vi "BLT-STATIC-CONFIG.vi"() -> ()   [LabVIEW 2018]
uses:
  Type Defs/Sensor Data.ctl
  Type Defs/Boxcar.ctl
panel:
  out "?":string="27.79 °C"
  out "?":string="27.79 °C"
  out "45% 2":string="27.79 °C"
  out "45%":string="27.79 °C"
  in  "Box cooler":bool
  out "NewVal":bool
  out "Ready To Fire Flag":bool
  out "Firing State":string[](array[string])=["System Is Not Armed", "", "", "", "", " "]
  in  "Arm Flag":bool
  in  "Sample Rate (secs)":u32=1000
  out "Burn Time\nCountdown (secs)":string="0.00"
  out "Boxcar Data":T1={"AI Sensor Data"={"Sensor Array"=[{"Description"="PT LOX Tank", "Last Reading"="1.37", "Coefs"=[0.0, 0.0], "Eng Units"="Psig"}, {"Description"="P3 - Fuel Tank Pressure", "Last Reading"="0.24", "Coefs"=[0.0, 5000.0], "Eng Units"="psig"}, {"Description"="P1 - Chamber Pressure", "Last Reading"="68.57", "Coefs"=[0.0, 5000.0], "Eng Units"="psig"}, {"Description"="Not Used", "Last Reading"="88.17", "Coefs"=[0.0, 0.0], "Eng Units"="psig"}, {"Description"="P5- DOME Reg.", "Last Reading"="1995.18", "Coefs"=[0.0, 5000.0], "Eng Units"="psig"}, {"Description"="Not Use", "Last Reading"="30.30", "Coefs"=[0.0, 0.0], "Eng Units"="psig"}, {"Description"="P4- High Pressure Tank", "Last Reading"="45.96", "Coefs"=[0.0, 10000.0], "Eng Units"="psig"}, {"Description"="P7 - Gnd High Pressure", "Last Reading"="1989.04", "Coefs"=[0.0, 10000.0], "Eng Units"="psig"}, {"Description"="P6 - GHE Fill Pressure", "Last Reading"="9918.82", "Coefs"=[0.0, 5000.0], "Eng Units"="psig"}, {"Description"="P8 - Pneumatics Pressure", "Last Reading"="9988.56", "Coefs"=[0.0, 5000.0], "Eng Units"="psig"}, {"Description"="Not Used", "Last Reading"="9997.25", "Coefs"=[0.0, 0.0], "Eng Units"=""}, {"Description"="Not Used", "Last Reading"="9988.56", "Coefs"=[0.0, 0.0], "Eng Units"=""}, {"Description"="Not Used", "Last Reading"="9948.58", "Coefs"=[0.0, 0.0], "Eng Units"=""}, {"Description"="Not Used", "Last Reading"="9973.45", "Coefs"=[0.0, 0.0], "Eng Units"=""}, {"Description"="Not Used", "Last Reading"="9964.45", "Coefs"=[0.0, 0.0], "Eng Units"=""}, {"Description"="PT High Press", "Last Reading"="9.16", "Coefs"=[0.0, 0.0], "Eng Units"="Psig"}, {"Description"="QD Sep Indication", "Last Reading"="2374.97", "Coefs"=[0.0, 1.0], "Eng Units"="On/Off"}, {"Description"="Lift Off Indicator", "Last Reading"="2375.24", "Coefs"=[0.0, 1.0], "Eng Units"="On/Off"}, {"Description"="Main Valve Open Indicator", "Last Reading"="2376.46", "Coefs"=[0.0, 1.0], "Eng Units"="On/Off"}, {"Description"="Main Valve Closed Indicator", "Last Reading"="2376.23", "Coefs"=[0.0, 1.0], "Eng Units"="On/Off"}, {"Description"="Load Cell 1 - Veh Gross Weight", "Last Reading"="2374.97", "Coefs"=[-122.0, 8333.3], "Eng Units"="lbf"}, {"Description"="Load Cell 2 - - Veh Gross Weight", "Last Reading"="2374.97", "Coefs"=[0.0, 8333.33], "Eng Units"="lbf"}, {"Description"="Not Used", "Last Reading"="2374.97", "Coefs"=[0.0, 0.0], "Eng Units"=""}, {"Description"="Not Used", "Last Reading"="2374.97", "Coefs"=[0.0, 0.0], "Eng Units"=""}, {"Description"="PT Fuel Tank", "Last Reading"="10.72", "Coefs"=[], "Eng Units"="Psig"}, {"Description"="", "Last Reading"="2401.98", "Coefs"=[], "Eng Units"=""}, {"Description"="PT Dome Set", "Last Reading"="0", "Coefs"=[], "Eng Units"="Psig"}, {"Description"="", "Last Reading"="2402.71", "Coefs"=[], "Eng Units"=""}, {"Description"="", "Last Reading"="2402.21", "Coefs"=[], "Eng Units"=""}, {"Description"="", "Last Reading"="2401.71", "Coefs"=[], "Eng Units"=""}, {"Description"="", "Last Reading"="2401.48", "Coefs"=[], "Eng Units"=""}, {"Description"="", "Last Reading"="2400.99", "Coefs"=[], "Eng Units"=""}]}, "TC Array"=[27.792357874999993, 27.792357874999993, 27.792357874999993, 27.792357874999993, 27.792357874999993, 27.792357874999993, 27.792357874999993, 1369.6815, 1369.6815, 1369.6815, 1369.6815, 1369.6815, 1369.6815, 1369.6815]}
  out "?":string="3.07 psig"
  out "Log Refnum":refnum<file>
  out "Log Epoch":u32
  out "Log Number":i32=8
  in  "Data Log Flag":bool
  out "File Path":path
  out "Eng Data & Units":string[](array[string])
  out "TC String Array":string[](array[string])=["27.79 °C", "27.79 °C", "27.79 °C", "27.79 °C", "27.79 °C", "27.79 °C", "27.79 °C", "1369.68 °C", "1369.68 °C", "1369.68 °C", "1369.68 °C", "1369.68 °C", "1369.68 °C", "1369.68 °C"]
  in  "Data Log Button":bool
  in  "Sequence Abort":bool
  out "Igniter Abort":bool
  out "Elapsed Time":u32=10554
  in  "Auto Sequence":bool
  in  "Auto Sequence Flag":bool
  out "Epoch":u32=5746771
  out "Countdown (secs)":i32
  in  "MV Open Start":dbl
  in  "Burn Time":dbl=10.0
  in  "Igniter Start":dbl=-3.0
  in  "Countdown":dbl=-10.0
  in  "Igniter Minimum\nTemp (°C)":dbl=200.0
  in  "Auto Switch":bool=TRUE
  out "?":string="1369.68 °C"
  out "Thermometer 2":dbl(slide)=1369.6815 scale=0.0..1000.0
  out "Thermometer":dbl(slide)=1369.6815 scale=0.0..1000.0
  out "Igniter Temp (°C)":string="1369.68 °C"
  out "?":string="27.79 °C"
  out "30%":string="27.79 °C"
  out "QD Sep Indicator":bool=TRUE
  out "Liftoff Indicator":bool=TRUE
  out "MV Closed Ind":bool
  out "MV Open Ind":bool
  out "?":string="0.13 lbf"
  out "?":string="0.32 psig"
  out "?":string="-4.62 psig"
  out "Dome Set PT":string="-1.58 psig"
  out "High Press PT":string="-1.56 psig"
  out "?":string="-1.17 psig"
  out "FUEL Tank PT":string="-1.03 psig"
  in  "High Press":bool
  in  "High Press Vent":bool
  in  "MV Open":bool
  in  "MV Closed":bool
  out "LOX Tank PT":string="-1.67 psig"
  in  "Remote QD Sep":bool
  in  "GHe Fill":bool
  in  "Igniter Pwr":bool
  in  "Dome Reg":bool
  in  "Dome Vent":bool
  in  "Fuel Vent":bool
  in  "LOX Vent":bool
  out "Relay States":bool[](array[boolean])
  in  "stop":bool
  in  "AI Sensor Data":T2={"Sensor Array"=[{"Description"="PT LOX Tank", "Last Reading"="1.37", "Coefs"=[0.0, 0.0], "Eng Units"="Psig"}, {"Description"="P3 - Fuel Tank Pressure", "Last Reading"="0.24", "Coefs"=[0.0, 5000.0], "Eng Units"="psig"}, {"Description"="P1 - Chamber Pressure", "Last Reading"="68.57", "Coefs"=[0.0, 5000.0], "Eng Units"="psig"}, {"Description"="Not Used", "Last Reading"="88.17", "Coefs"=[0.0, 0.0], "Eng Units"="psig"}, {"Description"="P5- DOME Reg.", "Last Reading"="1995.18", "Coefs"=[0.0, 5000.0], "Eng Units"="psig"}, {"Description"="Not Use", "Last Reading"="30.30", "Coefs"=[0.0, 0.0], "Eng Units"="psig"}, {"Description"="P4- High Pressure Tank", "Last Reading"="45.96", "Coefs"=[0.0, 10000.0], "Eng Units"="psig"}, {"Description"="P7 - Gnd High Pressure", "Last Reading"="1989.04", "Coefs"=[0.0, 10000.0], "Eng Units"="psig"}, {"Description"="P6 - GHE Fill Pressure", "Last Reading"="9918.82", "Coefs"=[0.0, 5000.0], "Eng Units"="psig"}, {"Description"="P8 - Pneumatics Pressure", "Last Reading"="9988.56", "Coefs"=[0.0, 5000.0], "Eng Units"="psig"}, {"Description"="Not Used", "Last Reading"="9997.25", "Coefs"=[0.0, 0.0], "Eng Units"=""}, {"Description"="Not Used", "Last Reading"="9988.56", "Coefs"=[0.0, 0.0], "Eng Units"=""}, {"Description"="Not Used", "Last Reading"="9948.58", "Coefs"=[0.0, 0.0], "Eng Units"=""}, {"Description"="Not Used", "Last Reading"="9973.45", "Coefs"=[0.0, 0.0], "Eng Units"=""}, {"Description"="Not Used", "Last Reading"="9964.45", "Coefs"=[0.0, 0.0], "Eng Units"=""}, {"Description"="PT High Press", "Last Reading"="9.16", "Coefs"=[0.0, 0.0], "Eng Units"="Psig"}, {"Description"="QD Sep Indication", "Last Reading"="2374.97", "Coefs"=[0.0, 1.0], "Eng Units"="On/Off"}, {"Description"="Lift Off Indicator", "Last Reading"="2375.24", "Coefs"=[0.0, 1.0], "Eng Units"="On/Off"}, {"Description"="Main Valve Open Indicator", "Last Reading"="2376.46", "Coefs"=[0.0, 1.0], "Eng Units"="On/Off"}, {"Description"="Main Valve Closed Indicator", "Last Reading"="2376.23", "Coefs"=[0.0, 1.0], "Eng Units"="On/Off"}, {"Description"="Load Cell 1 - Veh Gross Weight", "Last Reading"="2374.97", "Coefs"=[-122.0, 8333.3], "Eng Units"="lbf"}, {"Description"="Load Cell 2 - - Veh Gross Weight", "Last Reading"="2374.97", "Coefs"=[0.0, 8333.33], "Eng Units"="lbf"}, {"Description"="Not Used", "Last Reading"="2374.97", "Coefs"=[0.0, 0.0], "Eng Units"=""}, {"Description"="Not Used", "Last Reading"="2374.97", "Coefs"=[0.0, 0.0], "Eng Units"=""}, {"Description"="PT Fuel Tank", "Last Reading"="10.72", "Coefs"=[], "Eng Units"="Psig"}, {"Description"="", "Last Reading"="2401.98", "Coefs"=[], "Eng Units"=""}, {"Description"="PT Dome Set", "Last Reading"="0", "Coefs"=[], "Eng Units"="Psig"}, {"Description"="", "Last Reading"="2402.71", "Coefs"=[], "Eng Units"=""}, {"Description"="", "Last Reading"="2402.21", "Coefs"=[], "Eng Units"=""}, {"Description"="", "Last Reading"="2401.71", "Coefs"=[], "Eng Units"=""}, {"Description"="", "Last Reading"="2401.48", "Coefs"=[], "Eng Units"=""}, {"Description"="", "Last Reading"="2400.99", "Coefs"=[], "Eng Units"=""}]}
  # "CSULB Launch Team Control System"
  # "Questions regrads this system please direct them to Thanh Truc Le truclee126@gmail.com"
  # "Autosequence\n Parameters"
  # "TOP"
  # "TOP"
  # "CENTER"
  # "CENTER"
  # "BOTTOM"
  # "BOTTOM"
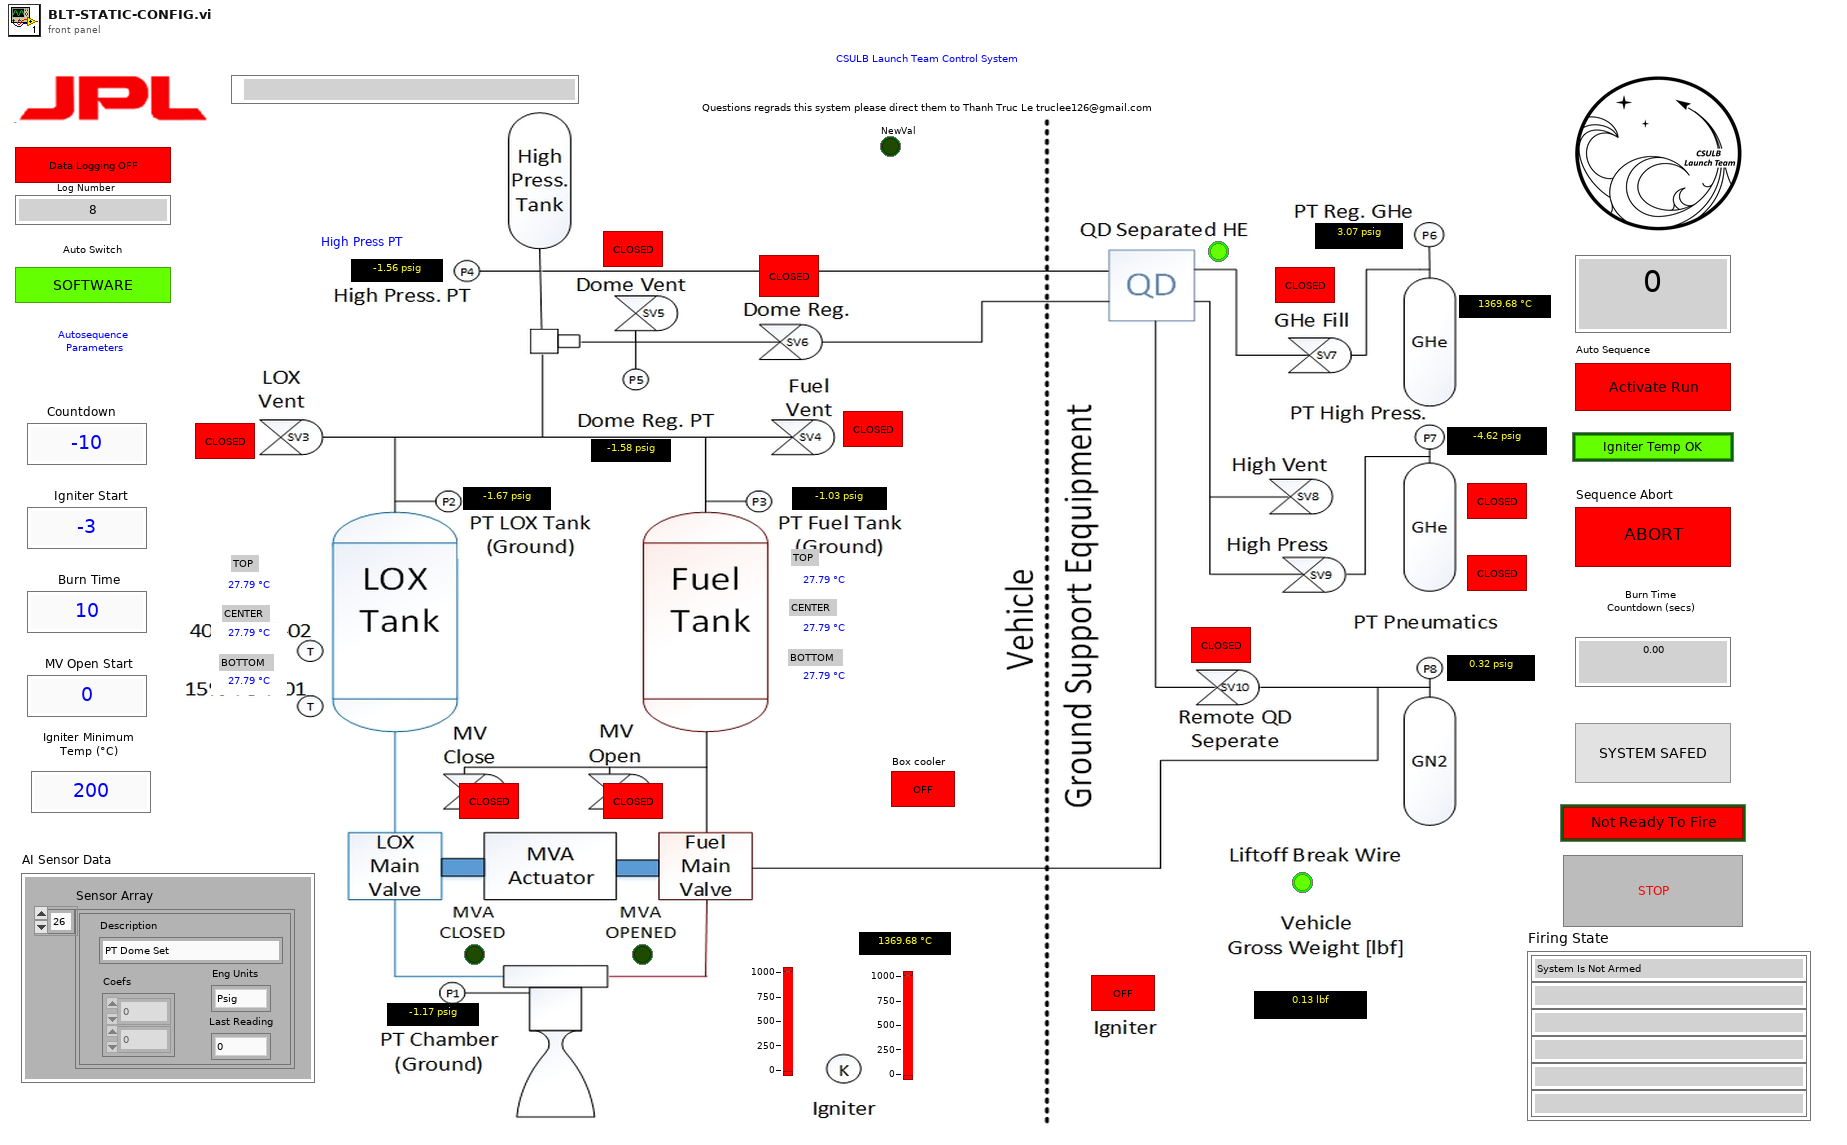
[diagram p1: front panel]
types:
  T1 = typedef "Boxcar.ctl" = cluster{"AI Sensor Data":T2, "TC Array":dbl[]}
  T2 = typedef "Sensor Data.ctl" = cluster{"Sensor Array":cluster{"Description":string, "Last Reading":string, "Coefs":dbl[], "Eng Units":string}[]}
  T3 = cluster{"Description":string, "Last Reading":string, "Coefs":dbl[], "Eng Units":string}[]
  T4 = enum16{"open", "replace", "create", "open or create", "replace or create", "replace or create with confirmation"}
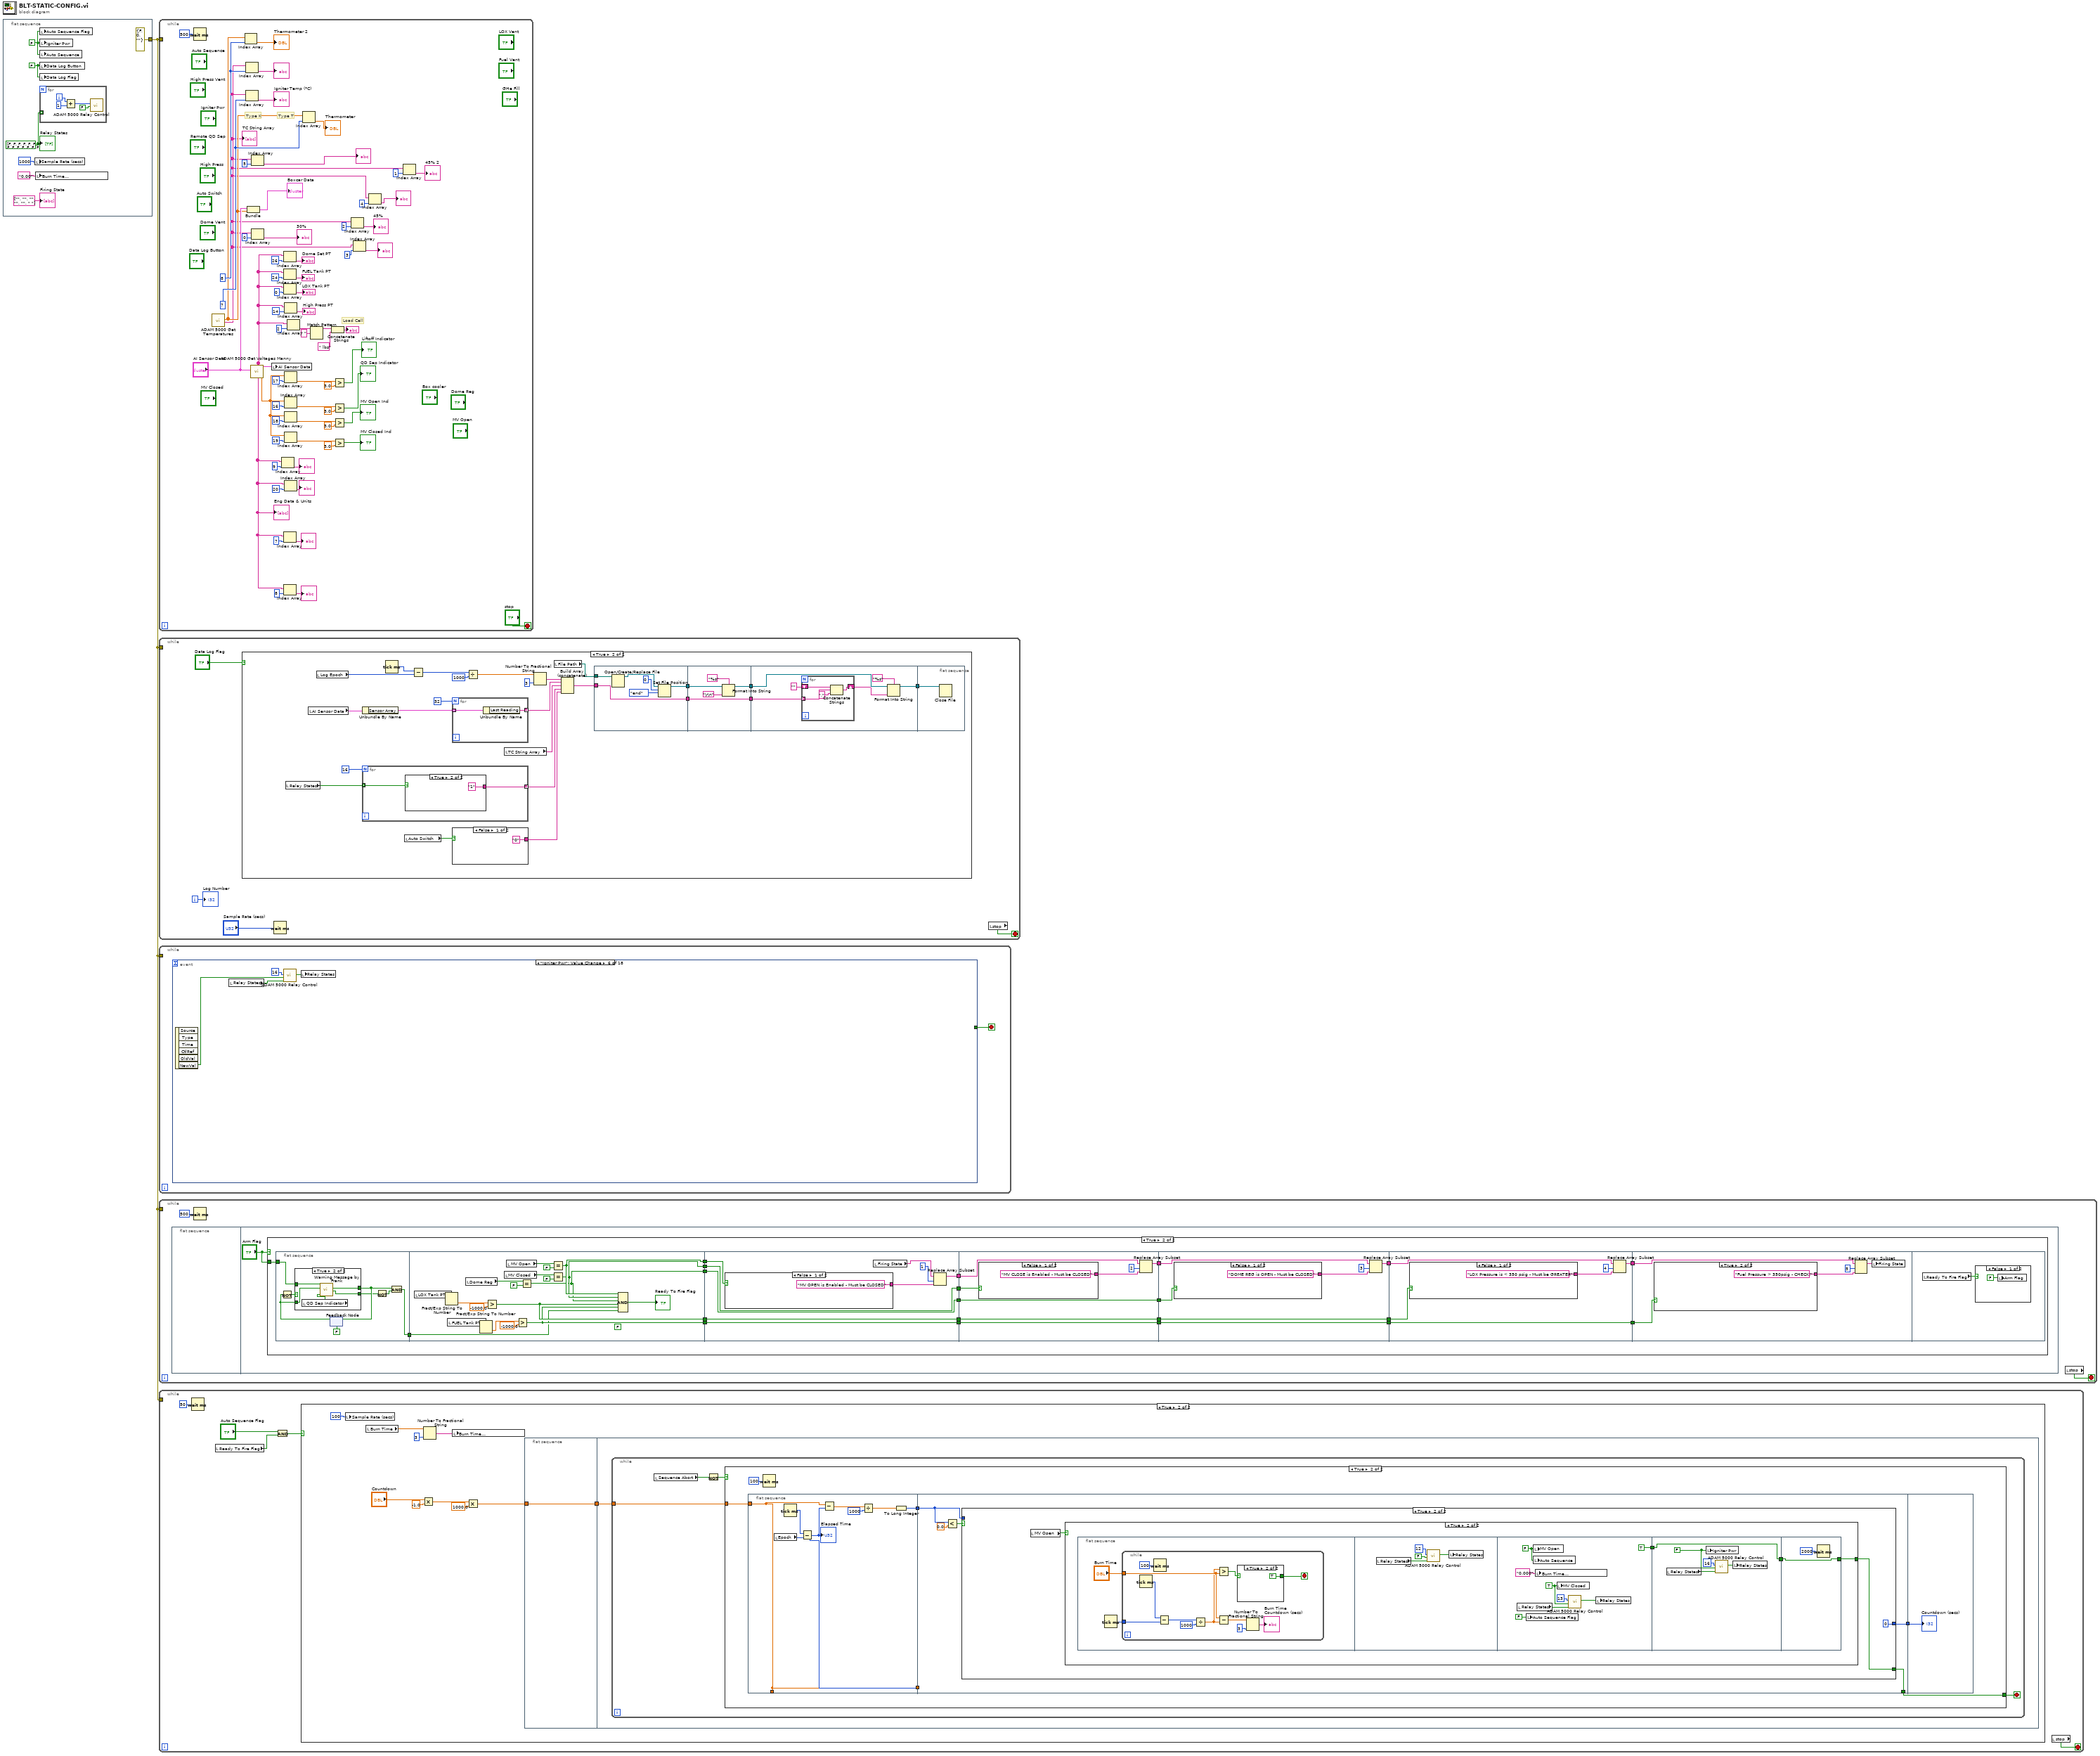
[diagram p0: block diagram]
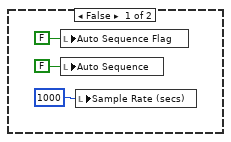
[diagram p2: hidden frame]
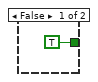
[diagram p3: hidden frame]
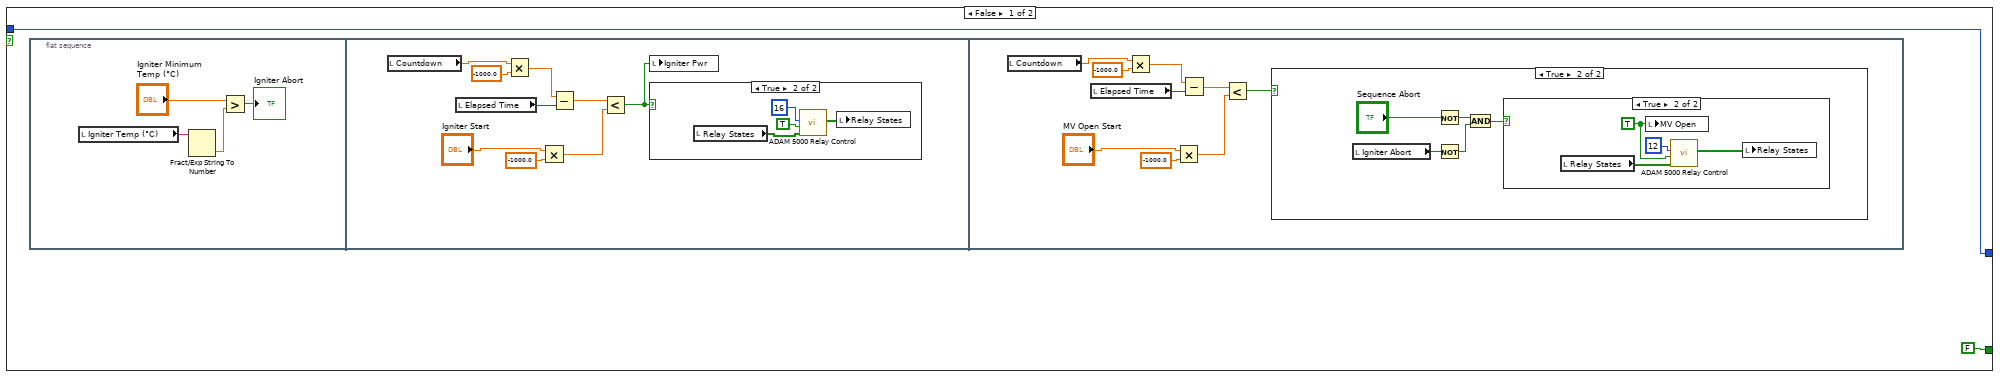
[diagram p4: hidden frame]
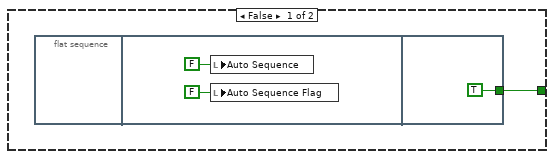
[diagram p8: hidden frame]
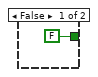
[diagram p9: hidden frame]
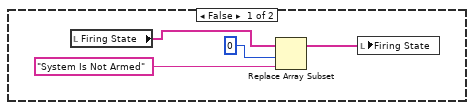
[diagram p10: hidden frame]
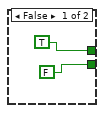
[diagram p11: hidden frame]
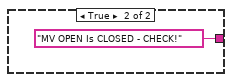
[diagram p12: hidden frame]
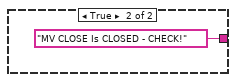
[diagram p13: hidden frame]
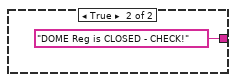
[diagram p14: hidden frame]
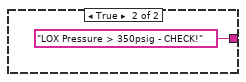
[diagram p15: hidden frame]
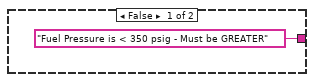
[diagram p16: hidden frame]
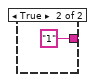
[diagram p19: hidden frame]
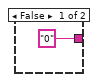
[diagram p20: hidden frame]
diagram:
  n1 = flat-sequence {
    tunnel: [errorcluster {"status"=FALSE, "code"=0, "source"=""} ("error constant")] -> w1
    frame #0 {
      w5 = FALSE ("Data Lof Flag")
      w6 = FALSE ("Auto Sequence Flag")
      w7 = bool[] [FALSE, FALSE, FALSE, FALSE, FALSE, FALSE, FALSE, FALSE, FALSE, FALSE, FALSE, FALSE, FALSE, FALSE, FALSE, FALSE]
      n2 = local write "Sample Rate (secs)"(u32 1000 ("Sample Rate (secs)")) -> ()
      n3 = local write "Burn Time\nCountdown (secs)"("0.00" ("Burn Time\nCountdown (secs)")) -> ()
      n4 = local write "Auto Sequence Flag"(w6) -> ()
      n5 = local write "Igniter Pwr"(w6) -> ()
      n6 = local write "Auto Sequence"(w6) -> ()
      n7 = local write "Data Log Button"(w5) -> ()
      n8 = local write "Data Log Flag"(w5) -> ()
      n9 = for {
        tunnel: w7 -> [_] mode=indexing
        i -> [w12]
        n10 = Add(x=w12, y=1) -> (x+y=w10:i32)
        n11 = call "ADAM 5000 Relay Control.vi"("State"=FALSE, "Relay # (1=1st relay)"=w10) -> ()  [unwired: 9 in, 1 out]
      }
      "Relay States" <- w7
      "Firing State" <- string[] ["", "", "", "", "", " "]
    }
  }
  n12 = while {
    tunnel: w1 -> [_]
    stop <- "stop" stop-if-true
    w37 = 7 ("index")
    w34 = 8 ("index")
    # "Load Cell"
    # "Type T"
    # "Type K"
    n13 = Wait (ms)(milliseconds to wait=u32 500) -> ()  [unwired: 1 out]
    n14 = call "ADAM 5000 Get Temperatures.vi"() -> ("TC String Array"=w16:string[], "TC Array"=w28:dbl[])  [unwired: 10 in]
    "TC String Array" <- w16
    n15 = Index Array(array=w28, index=w34) -> (element=→"Thermometer 2":dbl)
    n16 = Index Array(array=w16, index=w34) -> (element=→"?":string)
    n17 = Index Array(array=w16, index=w37) -> (element=→"Igniter Temp (°C)":string)
    n18 = Bundle("AI Sensor Data"="AI Sensor Data", "TC Array"=w28) -> (→"Boxcar Data":cluster{"AI Sensor Data":T2, "TC Array":dbl[]})  [unwired: 1 in]
    n19 = call "ADAM 5000 Get Voltages Manny.vi"("AI Sensor Data"="AI Sensor Data") -> ("Master Raw Data Vdc"=w43:dbl[], "AI Sensor Data Out"=w75:T2, "Eng Data & Units"=w30:string[])  [unwired: 5 in, 3 out]
    "Eng Data & Units" <- w30
    n20 = Index Array(array=w16, index=5) -> (element=→"?":string)
    n21 = Index Array(array=w16, index=0) -> (element=→"30%":string)
    n22 = local write "AI Sensor Data"(w75) -> ()
    n23 = Index Array(array=w30, index=9) -> (element=→"?":string)
    n24 = Index Array(array=w30, index=26) -> (element=→"Dome Set PT":string)
    n25 = Index Array(array=w30, index=24) -> (element=→"FUEL Tank PT":string)
    n26 = Index Array(array=w30, index=7) -> (element=→"?":string)
    n27 = Index Array(array=w30, index=0) -> (element=→"LOX Tank PT":string)
    n28 = Index Array(array=w30, index=8) -> (element=→"?":string)
    n29 = Index Array(array=w30, index=14) -> (element=→"High Press PT":string)
    n30 = Index Array(array=w43, index=17) -> (element=w50:dbl)
    n31 = Index Array(array=w43, index=16) -> (element=w45:dbl)
    n32 = Index Array(array=w43, index=18) -> (element=w58:dbl)
    n33 = Index Array(array=w43, index=19) -> (element=w54:dbl)
    n34 = Index Array(array=w30, index=20) -> (element=→"?":string)
    n35 = Index Array(array=w30, index=2) -> (element=w22:string)
    n36 = Index Array(array=w28, index=w37) -> (element=→"Thermometer":dbl)
    n37 = Match Pattern(string=w22, regular expression=" ") -> (before substring=w20:string)  [unwired: 1 in, 3 out]
    n38 = Concatenate Strings(w20, " lbs" ("string")) -> (→"?":string)
    n39 = Greater?(x=w50, y=3.0) -> (0:→"Liftoff Indicator":bool)
    n40 = Greater?(x=w45, y=3.0) -> (0:→"QD Sep Indicator":bool)
    n41 = Greater?(x=w58, y=3.0) -> (0:→"MV Open Ind":bool)
    n42 = Greater?(x=w54, y=3.0) -> (0:→"MV Closed Ind":bool)
    n43 = Index Array(array=w16, index=2) -> (element=→"45%":string)
    n44 = Index Array(array=w16, index=3) -> (element=→"?":string)
    n45 = Index Array(array=w16, index=4) -> (element=→"?":string)
    n46 = Index Array(array=w16, index=1) -> (element=→"45% 2":string)
  }
  n47 = while {
    tunnel: w1 -> [_]
    i -> [w79]
    stop <- w81 stop-if-true
    n48 = case shown="True" "Data Log Flag" {
      frame False {
      }
      frame True {
        n49 = local read "Relay States"() -> (w103:bool[])
        n50 = local read "AI Sensor Data"() -> (w105:T2)
        n51 = local read "Log Epoch"() -> (w96:u32)
        n52 = Unbundle By Name(w105) -> ("Sensor Array"=w104:T3)
        n53 = for {
          N: 16 -> [_]
          tunnel: w103 -> [w131] mode=indexing
          tunnel: [w130] -> w99 mode=indexing
          n54 = case shown="True" w131 {
            tunnel: ["0" "1"] -> w130
            frame False {
            }
            frame True {
            }
          }
        }
        n55 = Tick Count (ms)() -> (millisecond timer value=w97:u32)
        n56 = local read "Auto Switch"() -> (w102:bool)
        n57 = Subtract(x=w97, y=w96) -> (x-y=w95:u32)
        n58 = for {
          N: 32 -> [_]
          tunnel: w104 -> [w135] mode=indexing
          tunnel: [w134] -> w101 mode=indexing
          n59 = Unbundle By Name(w135) -> ("Last Reading"=w134:string)
        }
        n60 = case shown="False" w102 {
          tunnel: ["0" "1"] -> w98
          frame False {
          }
          frame True {
          }
        }
        n61 = Divide(x=w95, y=u32 1000) -> (x/y=w93:dbl)
        n62 = local read "TC String Array"() -> (w100:string[])
        n63 = Number To Fractional String(number=w93, precision (6)=i16 3) -> (F-format string=w91:string)  [unwired: 2 in]
        n64 = local read "File Path"() -> (w90:path)
        n65 = Build Array (concatenate)(w91, w101, w100, w99, w98) -> (w89:string[])
        n66 = flat-sequence {
          tunnel: w89 -> [w111]
          tunnel: w90 -> [w110]
          tunnel: [w111] -> w87
          tunnel: [w106] -> w84
          tunnel: [w112] -> w88
          tunnel: w87 -> [w116]
          tunnel: [w116] -> w86
          tunnel: w84 -> [w113]
          tunnel: w88 -> [w119]
          tunnel: w86 -> [w122]
          tunnel: [w117] -> w85
          tunnel: w85 -> [w127]
          frame #0 {
            n67 = Open/Create/Replace File(file path (use dialog)=w110) -> (refnum out=w109:refnum<file>)  [unwired: 5 in, 2 out]
            n68 = Set File Position(offset (in bytes) (0)=i64 0, refnum=w109, from (0:start)=enum16{"start", "end", "current"}."end") -> (refnum out=w106:refnum<file>)  [unwired: 1 in, 1 out]
          }
          frame #1 {
            n69 = Format Into String(format string="%s", initial string=w113, "\r\n") -> (resulting string=w112:refnum<file>)  [unwired: 1 in, 1 out]
          }
          frame #2 {
            n70 = for {
              shift-right: [w124] -> w118
              shift-left: "" -> [w123]
              tunnel: w122 -> [w126] mode=indexing
              n71 = Concatenate Strings(w123, w126, "," ("string")) -> (w124:string)
            }
            n72 = Format Into String(format string="%s", initial string=w119, w118) -> (resulting string=w117:refnum<file>)  [unwired: 1 in, 1 out]
          }
          frame #3 {
            n73 = Close File(refnum=w127) -> ()  [unwired: 1 in, 2 out]
          }
        }
      }
    }
    n74 = Wait (ms)(milliseconds to wait="Sample Rate (secs)") -> ()  [unwired: 1 out]
    n75 = local read "stop"() -> (w81:bool)
    "Log Number" <- w79
  }
  n76 = while {
    tunnel: w1 -> [_]
    stop <- w136 stop-if-true
    n77 = event shown="[5] \"Igniter Pwr\": Value Change" {
      selector: _ -> [_ _ _ _ _ _ _ _ _ _ _ _ _ _ _ _ _ _]
      dyn-events: _ -> [_ _ _ _ _ _ _ _ _ _ _ _ _ _ _ _ _ _]
      timeout: _ -> [_ _ _ _ _ _ _ _ _ _ _ _ _ _ _ _ _ _]
      tunnel: [_ _ _ _ _ _ _ _ w165 _ _ _ _ _ _ _ _ _] -> w136
      event Timeout {
        n78 = event-data() -> ()  [unwired: 1 in, 3 out]
      }
      event "LOX Vent": Value Change {
        n79 = event-data() -> ("NewVal"=w139:bool)  [unwired: 1 in, 5 out]
        n80 = local read "Relay States"() -> (w138:bool[])
        n81 = call "ADAM 5000 Relay Control.vi"("Relay States IN"=w138, "State"=w139, "Relay # (1=1st relay)"=1) -> ("Relay States OUT"=w137:bool[])  [unwired: 8 in]
        n82 = local write "Relay States"(w137) -> ()
      }
      event "Fuel Vent": Value Change {
        n83 = event-data() -> ("NewVal"=w141:bool)  [unwired: 1 in, 5 out]
        n84 = local read "Relay States"() -> (w143:bool[])
        n85 = call "ADAM 5000 Relay Control.vi"("Relay States IN"=w143, "State"=w141, "Relay # (1=1st relay)"=2) -> ("Relay States OUT"=w142:bool[])  [unwired: 8 in]
        n86 = local write "Relay States"(w142) -> ()
      }
      event "Dome Vent": Value Change {
        n87 = event-data() -> ("NewVal"=w145:bool)  [unwired: 1 in, 5 out]
        n88 = local read "Relay States"() -> (w147:bool[])
        n89 = call "ADAM 5000 Relay Control.vi"("Relay States IN"=w147, "State"=w145, "Relay # (1=1st relay)"=6) -> ("Relay States OUT"=w146:bool[])  [unwired: 8 in]
        n90 = local write "Relay States"(w146) -> ()
      }
      event "Dome Reg": Value Change {
        n91 = event-data() -> ("NewVal"=w149:bool)  [unwired: 1 in, 5 out]
        n92 = local read "Relay States"() -> (w151:bool[])
        n93 = call "ADAM 5000 Relay Control.vi"("Relay States IN"=w151, "State"=w149, "Relay # (1=1st relay)"=5) -> ("Relay States OUT"=w150:bool[])  [unwired: 8 in]
        n94 = local write "Relay States"(w150) -> ()
      }
      event "Igniter Pwr": Value Change {
        n95 = event-data() -> ("NewVal"=w153:bool)  [unwired: 1 in, 5 out]
        n96 = local read "Relay States"() -> (w155:bool[])
        n97 = call "ADAM 5000 Relay Control.vi"("Relay States IN"=w155, "State"=w153, "Relay # (1=1st relay)"=16) -> ("Relay States OUT"=w154:bool[])  [unwired: 8 in]
        n98 = local write "Relay States"(w154) -> ()
      }
      event "GHe Fill": Value Change {
        n99 = event-data() -> ("NewVal"=w157:bool)  [unwired: 1 in, 5 out]
        n100 = local read "Relay States"() -> (w159:bool[])
        n101 = call "ADAM 5000 Relay Control.vi"("Relay States IN"=w159, "State"=w157, "Relay # (1=1st relay)"=9) -> ("Relay States OUT"=w158:bool[])  [unwired: 8 in]
        n102 = local write "Relay States"(w158) -> ()
      }
      event "Remote QD Sep": Value Change {
        n103 = event-data() -> ("NewVal"=w161:bool)  [unwired: 1 in, 5 out]
        n104 = local read "Relay States"() -> (w163:bool[])
        n105 = call "ADAM 5000 Relay Control.vi"("Relay States IN"=w163, "State"=w161, "Relay # (1=1st relay)"=10) -> ("Relay States OUT"=w162:bool[])  [unwired: 8 in]
        n106 = local write "Relay States"(w162) -> ()
      }
      event "stop": Value Change {
        n107 = event-data() -> ()  [unwired: 1 in, 6 out]
        n108 = flat-sequence {
          tunnel: [TRUE] -> w165
          frame #0 {
            n109 = Wait (ms)(milliseconds to wait=u32 2000) -> ()  [unwired: 1 out]
          }
          frame #1 {
          }
        }
      }
      event "MV Closed": Value Change {
        n110 = event-data() -> ("NewVal"=w168:bool)  [unwired: 1 in, 5 out]
        n111 = local read "Relay States"() -> (w170:bool[])
        n112 = call "ADAM 5000 Relay Control.vi"("Relay States IN"=w170, "State"=w168, "Relay # (1=1st relay)"=13) -> ("Relay States OUT"=w169:bool[])  [unwired: 8 in]
        n113 = local write "Relay States"(w169) -> ()
      }
      event "High Press Vent": Value Change {
        n114 = event-data() -> ("NewVal"=w172:bool)  [unwired: 1 in, 5 out]
        n115 = local read "Relay States"() -> (w174:bool[])
        n116 = call "ADAM 5000 Relay Control.vi"("Relay States IN"=w174, "State"=w172, "Relay # (1=1st relay)"=15) -> ("Relay States OUT"=w173:bool[])  [unwired: 8 in]
        n117 = local write "Relay States"(w173) -> ()
      }
      event "High Press": Value Change {
        n118 = event-data() -> ("NewVal"=w176:bool)  [unwired: 1 in, 5 out]
        n119 = local read "Relay States"() -> (w178:bool[])
        n120 = call "ADAM 5000 Relay Control.vi"("Relay States IN"=w178, "State"=w176, "Relay # (1=1st relay)"=7) -> ("Relay States OUT"=w177:bool[])  [unwired: 8 in]
        n121 = local write "Relay States"(w177) -> ()
      }
      event "Auto Switch": Value Change {
        n122 = event-data() -> ("NewVal"=w181:bool)  [unwired: 1 in, 5 out]
        n123 = call "Control ETH008 Relay.vi"("On/Off"=w181, "Relay Number"=1) -> ()  [unwired: 10 in]
      }
      event "Auto Sequence": Value Change {
        w182 = TRUE ("Auto Sequence Flag")
        n124 = event-data() -> ()  [unwired: 1 in, 6 out]
        n125 = Tick Count (ms)() -> (millisecond timer value=→"Epoch":u32)
        n126 = local write "Auto Sequence Flag"(w182) -> ()
        n127 = local write "Auto Sequence"(w182) -> ()
      }
      event "Sequence Abort": Value Change {
        n128 = event-data() -> ()  [unwired: 1 in, 6 out]
        n129 = flat-sequence {
          frame #0 {
            w184 = FALSE ("Auto Sequence Flag")
            n130 = local write "Auto Sequence Flag"(w184) -> ()
            n131 = local write "Igniter Pwr"(w184) -> ()
            n132 = local write "Auto Sequence"(w184) -> ()
          }
          frame #1 {
            n133 = for {
              tunnel: bool[] [FALSE, FALSE, FALSE, FALSE, FALSE, FALSE, FALSE, FALSE, FALSE, FALSE, FALSE, FALSE, FALSE, FALSE, FALSE, FALSE] -> [_] mode=indexing
              i -> [w189]
              n134 = Add(x=w189, y=1) -> (x+y=w187:i32)
              n135 = call "ADAM 5000 Relay Control.vi"("State"=FALSE, "Relay # (1=1st relay)"=w187) -> ()  [unwired: 9 in, 1 out]
            }
          }
        }
      }
      event "Data Log Button": Value Change {
        n136 = event-data() -> ("NewVal"=w190:bool)  [unwired: 1 in, 5 out]
        n137 = case shown="True" w190 {
          frame False {
            n138 = local write "Data Log Flag"(FALSE ("Data Lof Flag")) -> ()
            n139 = local write "Data Log Flag"(FALSE ("Data Lof Flag")) -> ()
            n140 = local write "Data Log Flag"(FALSE ("Data Lof Flag")) -> ()
            n141 = local write "Data Log Flag"(FALSE ("Data Lof Flag")) -> ()
            n142 = local write "Data Log Flag"(FALSE ("Data Lof Flag")) -> ()
            n143 = local write "Data Log Flag"(FALSE ("Data Lof Flag")) -> ()
            n144 = local write "Data Log Flag"(FALSE ("Data Lof Flag")) -> ()
            n145 = local write "Data Log Flag"(FALSE ("Data Lof Flag")) -> ()
            n146 = local write "Data Log Flag"(FALSE ("Data Lof Flag")) -> ()
            n147 = local write "Data Log Flag"(FALSE ("Data Lof Flag")) -> ()
            n148 = local write "Data Log Flag"(FALSE ("Data Lof Flag")) -> ()
          }
          frame True {
            n149 = flat-sequence {
              frame #0 {
                n150 = Tick Count (ms)() -> (millisecond timer value=→"Log Epoch":u32)
                n151 = for {
                  N: 14 -> [_]
                  tunnel: [w234] -> w213 mode=indexing
                  i -> [w233]
                  n152 = Add(x=w233, y=1) -> (x+y=w231:i32)
                  n153 = Number To Fractional String(number=w231, precision (6)=i16 0) -> (F-format string=w235:string)  [unwired: 2 in]
                  n154 = Concatenate Strings("TC", w235) -> (w234:string)
                }
                n155 = for {
                  N: 16 -> [_]
                  tunnel: [w227] -> w212 mode=indexing
                  i -> [w226]
                  n156 = Add(x=w226, y=1) -> (x+y=w224:i32)
                  n157 = Number To Fractional String(number=w224, precision (6)=i16 0) -> (F-format string=w228:string)  [unwired: 2 in]
                  n158 = Concatenate Strings("Relay", w228) -> (w227:string)
                }
                n159 = local read "AI Sensor Data"() -> (w219:T2)
                n160 = Unbundle By Name(w219) -> ("Sensor Array"=w218:T3)
                n161 = for {
                  tunnel: w218 -> [w239] mode=indexing
                  tunnel: [w238] -> w216 mode=indexing
                  n162 = Unbundle By Name(w239) -> ("Description"=w238:string)
                }
                n163 = Build Array (concatenate)("Time (s)", w216, w213, w212, "Manual/Auto (1=Auto)") -> (w208:string[])
                n164 = for {
                  shift-right: [w221] -> w206
                  shift-left: "" -> [w220]
                  tunnel: w208 -> [w223] mode=indexing
                  n165 = Concatenate Strings(w220, w223, "," ("string")) -> (w221:string)
                }
                n166 = Open/Create/Replace File(operation (0:open)=T4."replace or create") -> (refnum out=w205:refnum<file>)  [unwired: 5 in, 2 out]
                "Log Refnum" <- w205
                n167 = Refnum to Path(1:w205) -> (0:→"File Path":path)
                n168 = Format Into String(format string="%s", initial string=w205, w206) -> (resulting string=w202:refnum<file>)  [unwired: 1 in, 1 out]
                n169 = Close File(refnum=w202) -> ()  [unwired: 1 in, 2 out]
              }
              frame #1 {
                n170 = Wait (ms)(milliseconds to wait=u32 1000) -> ()  [unwired: 1 out]
              }
              frame #2 {
                n171 = local write "Data Log Flag"(TRUE ("Data Lof Flag")) -> ()
              }
            }
          }
        }
      }
      event "MV Open": Value Change {
        n172 = event-data() -> ("NewVal"=w245:bool)  [unwired: 1 in, 5 out]
        "NewVal" <- w245
        n173 = local read "Relay States"() -> (w243:bool[])
        n174 = call "ADAM 5000 Relay Control.vi"("Relay States IN"=w243, "State"=w245, "Relay # (1=1st relay)"=12) -> ("Relay States OUT"=w244:bool[])  [unwired: 8 in]
        n175 = local write "Relay States"(w244) -> ()
      }
      event "Box cooler": Value Change {
        n176 = event-data() -> ("NewVal"=w246:bool)  [unwired: 1 in, 5 out]
        n177 = local read "Relay States"() -> (w248:bool[])
        n178 = call "ADAM 5000 Relay Control.vi"("Relay States IN"=w248, "State"=w246, "Relay # (1=1st relay)"=3) -> ("Relay States OUT"=w249:bool[])  [unwired: 8 in]
        n179 = local write "Relay States"(w249) -> ()
      }
    }
  }
  n180 = while {
    tunnel: w1 -> [_]
    stop <- w250 stop-if-true
    n181 = flat-sequence {
      frame #0 {
      }
      frame #1 {
        n182 = case shown="True" "Arm Flag" {
          tunnel: "Arm Flag" -> [_ w258]
          frame False {
            n183 = local read "Firing State"() -> (w256:string[])
            n184 = Replace Array Subset(array=w256, new element="System Is Not Armed" ("new element/subarray"), index=0) -> (w253:string[])
            n185 = local write "Firing State"(w253) -> ()
          }
          frame True {
            n186 = flat-sequence {
              tunnel: w258 -> [w281]
              tunnel: [w279] -> w257
              tunnel: [w299] -> w277
              tunnel: [w298] -> w275
              tunnel: [w297] -> w271
              tunnel: [w296] -> w265
              tunnel: [w295] -> w260
              tunnel: w257 -> [w294]
              tunnel: w277 -> [w320]
              tunnel: [w316] -> w276
              tunnel: w275 -> [w316]
              tunnel: [w315] -> w274
              tunnel: [w314] -> w272
              tunnel: w271 -> [w314]
              tunnel: [w313] -> w266
              tunnel: w265 -> [w313]
              tunnel: [w312] -> w261
              tunnel: w260 -> [w312]
              tunnel: w276 -> [w328]
              tunnel: w274 -> [w327]
              tunnel: [w326] -> w273
              tunnel: w272 -> [w326]
              tunnel: [w325] -> w270
              tunnel: [w324] -> w267
              tunnel: w266 -> [w324]
              tunnel: [w323] -> w262
              tunnel: w261 -> [w323]
              tunnel: w273 -> [w337]
              tunnel: w270 -> [w336]
              tunnel: [w335] -> w269
              tunnel: [w334] -> w268
              tunnel: w267 -> [w334]
              tunnel: [w333] -> w263
              tunnel: w262 -> [w333]
              tunnel: w269 -> [w345]
              tunnel: w268 -> [w344]
              tunnel: [w343] -> w264
              tunnel: w263 -> [w343]
              tunnel: [w342] -> w259
              tunnel: w264 -> [w352]
              tunnel: w259 -> [w351]
              frame #0 {
                n187 = feedback #1(FALSE) -> (w280:bool)
                n188 = Not(x=w280) -> (.not. x?=w285:bool)
                n189 = case shown="True" w285 {
                  tunnel: [TRUE w292] -> w284
                  tunnel: [FALSE w291] -> w283
                  tunnel: w281 -> [_ w290]
                  tunnel: w280 -> [_ w288]
                  frame False {
                  }
                  frame True {
                    n190 = local read "QD Sep Indicator"() -> (w289:bool)
                    n191 = call "Warning Message by Frank.vi"("Contiuous"=w289, "ok?"=w288, "Arm Flag"=w290) -> ("super cancel"=w291:bool, "super ok"=w292:bool)  [unwired: 6 in, 1 out]
                  }
                }
                n192 = feedback-in #1(w284) -> ()
                n193 = Not(x=w283) -> (.not. x?=w282:bool)
                n194 = And(x=w284, y=w282) -> (x .and. y?=w279:bool)
              }
              frame #1 {
                (unwired) FALSE ("x .and. y?")
                n195 = local read "LOX Tank PT"() -> (w305:string)
                n196 = Fract/Exp String To Number(string=w305) -> (number=w304:dbl)  [unwired: 3 in, 1 out]
                n197 = local read "FUEL Tank PT"() -> (w300:string)
                n198 = local read "Dome Reg"() -> (w307:bool)
                n199 = Fract/Exp String To Number(string=w300) -> (number=w301:dbl)  [unwired: 3 in, 1 out]
                n200 = Greater?(x=w304, y=-1000.0) -> (0:w296:bool)
                n201 = local read "MV Closed"() -> (w308:bool)
                n202 = local read "MV Open"() -> (w311:bool)
                n203 = Greater?(x=w301, y=-1000.0) -> (0:w295:bool)
                n204 = Equal?(x=w307, y=FALSE) -> (x = y?=w297:bool)
                n205 = Equal?(x=w311, y=FALSE) -> (x = y?=w299:bool)
                n206 = Equal?(x=w308, y=FALSE) -> (x = y?=w298:bool)
                n207 = Compound Arithmetic op=AND(w299, w298, w297, w296, w295, w294) -> (→"Ready To Fire Flag":bool)
              }
              frame #2 {
                n208 = case shown="False" w320 {
                  tunnel: ["MV OPEN is Enabled - Must be CLOSED" "MV OPEN Is CLOSED - CHECK!"] -> w317
                  frame False {
                  }
                  frame True {
                  }
                }
                n209 = local read "Firing State"() -> (w319:string[])
                n210 = Replace Array Subset(array=w319, new element=w317, index=1) -> (w315:string[])
              }
              frame #3 {
                n211 = case shown="False" w328 {
                  tunnel: ["MV CLOSE is Enabled - Must be CLOSED" "MV CLOSE Is CLOSED - CHECK!"] -> w330
                  frame False {
                  }
                  frame True {
                  }
                }
                n212 = Replace Array Subset(array=w327, new element=w330, index=2) -> (w325:string[])
              }
              frame #4 {
                n213 = case shown="False" w337 {
                  tunnel: ["DOME REG is OPEN - Must be CLOSED" "DOME Reg is CLOSED - CHECK!"] -> w338
                  frame False {
                  }
                  frame True {
                  }
                }
                n214 = Replace Array Subset(array=w336, new element=w338, index=3) -> (w335:string[])
              }
              frame #5 {
                n215 = case shown="False" w344 {
                  tunnel: ["LOX Pressure is < 350 psig - Must be GREATER" "LOX Pressure > 350psig - CHECK!"] -> w347
                  frame False {
                  }
                  frame True {
                  }
                }
                n216 = Replace Array Subset(array=w345, new element=w347, index=4) -> (w342:string[])
              }
              frame #6 {
                n217 = case shown="True" w352 {
                  tunnel: ["Fuel Pressure is < 350 psig - Must be GREATER" "Fuel Pressure > 350psig - CHECK!"] -> w353
                  frame False {
                  }
                  frame True {
                  }
                }
                n218 = Replace Array Subset(array=w351, new element=w353, index=5) -> (w350:string[])
                n219 = local write "Firing State"(w350) -> ()
              }
              frame #7 {
                n220 = local read "Ready To Fire Flag"() -> (w357:bool)
                n221 = case shown="False" w357 {
                  frame False {
                    n222 = local write "Arm Flag"(FALSE ("Arm Flag")) -> ()
                  }
                  frame True {
                  }
                }
              }
            }
          }
        }
      }
    }
    n223 = Wait (ms)(milliseconds to wait=u32 500) -> ()  [unwired: 1 out]
    n224 = local read "stop"() -> (w250:bool)
  }
  n225 = while {
    tunnel: w1 -> [_]
    stop <- w363 stop-if-true
    n226 = Wait (ms)(milliseconds to wait=u32 50) -> ()  [unwired: 1 out]
    n227 = local read "Ready To Fire Flag"() -> (w360:bool)
    n228 = And(x="Auto Sequence Flag", y=w360) -> (x .and. y?=w359:bool)
    n229 = case shown="True" w359 {
      frame False {
        n230 = local write "Auto Sequence Flag"(FALSE ("Auto Sequence Flag")) -> ()
        n231 = local write "Auto Sequence"(FALSE ("Auto Sequence Flag")) -> ()
        n232 = local write "Sample Rate (secs)"(u32 1000 ("Sample Rate (secs)")) -> ()
      }
      frame True {
        n233 = local write "Sample Rate (secs)"(u32 100 ("Sample Rate (secs)")) -> ()
        n234 = local read "Burn Time"() -> (w370:dbl)
        n235 = Multiply(x="Countdown", y=-1.0) -> (x*y=w371:dbl)
        n236 = Number To Fractional String(number=w370, precision (6)=i16 3) -> (F-format string=w368:string)  [unwired: 2 in]
        n237 = local write "Burn Time\nCountdown (secs)"(w368) -> ()
        n238 = Multiply(x=w371, y=1000.0) -> (x*y=w375:dbl)
        n239 = flat-sequence {
          tunnel: w375 -> [w377]
          tunnel: [w377] -> w374
          tunnel: w374 -> [w378]
          frame #0 {
          }
          frame #1 {
            n240 = while {
              tunnel: w378 -> [w382]
              stop <- w381 stop-if-true
              n241 = local read "Sequence Abort"() -> (w380:bool)
              n242 = Not(x=w380) -> (.not. x?=w379:bool)
              n243 = case shown="True" w379 {
                tunnel: w382 -> [_ w386]
                tunnel: [TRUE w384] -> w381
                frame False {
                }
                frame True {
                  n244 = flat-sequence {
                    tunnel: [w393] -> _
                    tunnel: w386 -> [w393]
                    tunnel: [w394] -> w390
                    tunnel: [w393] -> w389
                    tunnel: [w391] -> w388
                    tunnel: w390 -> [_]
                    tunnel: w389 -> [_]
                    tunnel: w388 -> [w400]
                    tunnel: [w402] -> w384
                    tunnel: [w399] -> w387
                    tunnel: w387 -> [w486]
                    frame #0 {
                      n245 = local read "Epoch"() -> (w392:u32)
                      n246 = Tick Count (ms)() -> (millisecond timer value=w398:u32)
                      n247 = Subtract(x=w398, y=w392) -> (x-y=w394:u32)
                      "Elapsed Time" <- w394
                      n248 = Subtract(x=w393, y=w394) -> (x-y=w395:dbl)
                      n249 = Divide(x=w395, y=u32 1000) -> (x/y=w396:dbl)
                      n250 = To Long Integer(number=w396) -> (32bit integer=w391:i32)
                    }
                    frame #1 {
                      n251 = Less?(x=w400, y=0.0) -> (x < y?=w401:bool)
                      n252 = case shown="True" w401 {
                        tunnel: [FALSE w443] -> w402
                        tunnel: w400 -> [w404 _]
                        tunnel: [w404 0] -> w399
                        frame False {
                          n253 = flat-sequence {
                            frame #0 {
                              n254 = local read "Igniter Temp (°C)"() -> (w409:string)
                              n255 = Fract/Exp String To Number(string=w409) -> (number=w408:dbl)  [unwired: 3 in, 1 out]
                              n256 = Greater?(x="Igniter Minimum\nTemp (°C)", y=w408) -> (0:→"Igniter Abort":bool)
                            }
                            frame #1 {
                              n257 = local read "Countdown"() -> (w418:dbl)
                              n258 = local read "Elapsed Time"() -> (w415:u32)
                              n259 = Multiply(x=w418, y=-1000.0) -> (x*y=w416:dbl)
                              n260 = Multiply(x="Igniter Start", y=-1000.0) -> (x*y=w411:dbl)
                              n261 = Subtract(x=w416, y=w415) -> (x-y=w412:dbl)
                              n262 = Less?(x=w412, y=w411) -> (x < y?=w410:bool)
                              n263 = local write "Igniter Pwr"(w410) -> ()
                              n264 = case shown="True" w410 {
                                frame False {
                                }
                                frame True {
                                n265 = local read "Relay States"() -> (w420:bool[])
                                n266 = call "ADAM 5000 Relay Control.vi"("Relay States IN"=w420, "State"=TRUE, "Relay # (1=1st relay)"=16) -> ("Relay States OUT"=w419:bool[])  [unwired: 8 in]
                                n267 = local write "Relay States"(w419) -> ()
                                }
                              }
                            }
                            frame #2 {
                              n268 = local read "Countdown"() -> (w425:dbl)
                              n269 = local read "Elapsed Time"() -> (w428:u32)
                              n270 = Multiply(x=w425, y=-1000.0) -> (x*y=w427:dbl)
                              n271 = Multiply(x="MV Open Start", y=-1000.0) -> (x*y=w431:dbl)
                              n272 = Subtract(x=w427, y=w428) -> (x-y=w430:dbl)
                              n273 = Less?(x=w430, y=w431) -> (x < y?=w423:bool)
                              n274 = case shown="True" w423 {
                                frame False {
                                }
                                frame True {
                                n275 = local read "Igniter Abort"() -> (w435:bool)
                                n276 = Not(x="Sequence Abort") -> (.not. x?=w434:bool)
                                n277 = Not(x=w435) -> (.not. x?=w433:bool)
                                n278 = And(x=w434, y=w433) -> (x .and. y?=w432:bool)
                                n279 = case shown="True" w432 {
                                frame False {
                                }
                                frame True {
                                w437 = TRUE ("State")
                                n280 = local read "Relay States"() -> (w439:bool[])
                                n281 = local write "MV Open"(w437) -> ()
                                n282 = call "ADAM 5000 Relay Control.vi"("Relay States IN"=w439, "State"=w437, "Relay # (1=1st relay)"=12) -> ("Relay States OUT"=w438:bool[])  [unwired: 8 in]
                                n283 = local write "Relay States"(w438) -> ()
                                }
                                }
                                }
                              }
                            }
                          }
                        }
                        frame True {
                          n284 = local read "MV Open"() -> (w441:bool)
                          n285 = case shown="True" w441 {
                            tunnel: [w444 w450] -> w443
                            frame False {
                              n286 = flat-sequence {
                                tunnel: [TRUE] -> w444
                                frame #0 {
                                }
                                frame #1 {
                                n287 = local write "Auto Sequence"(FALSE ("Auto Sequence Flag")) -> ()
                                n288 = local write "Auto Sequence Flag"(FALSE ("Auto Sequence Flag")) -> ()
                                }
                                frame #2 {
                                }
                              }
                            }
                            frame True {
                              n289 = flat-sequence {
                                tunnel: [TRUE] -> w449
                                tunnel: w449 -> [w483]
                                tunnel: [w483] -> w448
                                tunnel: [w485] -> w450
                                tunnel: w448 -> [w485]
                                frame #0 {
                                n290 = Tick Count (ms)() -> (millisecond timer value=w451:u32)
                                n291 = while {
                                tunnel: "Burn Time" -> [w457]
                                tunnel: w451 -> [w462]
                                stop <- w458 stop-if-true
                                n292 = Tick Count (ms)() -> (millisecond timer value=w463:u32)
                                n293 = Wait (ms)(milliseconds to wait=u32 100) -> ()  [unwired: 1 out]
                                n294 = Subtract(x=w463, y=w462) -> (x-y=w461:u32)
                                n295 = Divide(x=w461, y=u32 1000) -> (x/y=w456:dbl)
                                n296 = Greater?(x=w456, y=w457) -> (0:w459:bool)
                                n297 = Subtract(x=w457, y=w456) -> (x-y=w455:dbl)
                                n298 = case shown="True" w459 {
                                tunnel: [FALSE TRUE] -> w458
                                frame False {
                                }
                                frame True {
                                }
                                }
                                n299 = Number To Fractional String(number=w455, precision (6)=i16 3) -> (F-format string=→"Burn Time\nCountdown (secs)":string)  [unwired: 2 in]
                                }
                                }
                                frame #1 {
                                n300 = local read "Relay States"() -> (w469:bool[])
                                n301 = call "ADAM 5000 Relay Control.vi"("Relay States IN"=w469, "State"=FALSE, "Relay # (1=1st relay)"=12) -> ("Relay States OUT"=w470:bool[])  [unwired: 8 in]
                                n302 = local write "Relay States"(w470) -> ()
                                }
                                frame #2 {
                                w473 = FALSE ("Auto Sequence Flag")
                                w472 = TRUE ("State")
                                n303 = local read "Relay States"() -> (w476:bool[])
                                n304 = local write "Auto Sequence Flag"(FALSE ("Auto Sequence Flag")) -> ()
                                n305 = local write "MV Open"(w473) -> ()
                                n306 = local write "Auto Sequence"(w473) -> ()
                                n307 = local write "Burn Time\nCountdown (secs)"("0.000" ("Burn Time\nCountdown (secs)")) -> ()
                                n308 = local write "MV Closed"(w472) -> ()
                                n309 = call "ADAM 5000 Relay Control.vi"("Relay States IN"=w476, "State"=w472, "Relay # (1=1st relay)"=13) -> ("Relay States OUT"=w477:bool[])  [unwired: 8 in]
                                n310 = local write "Relay States"(w477) -> ()
                                }
                                frame #3 {
                                w479 = FALSE ("State")
                                n311 = local read "Relay States"() -> (w481:bool[])
                                n312 = local write "Igniter Pwr"(w479) -> ()
                                n313 = call "ADAM 5000 Relay Control.vi"("Relay States IN"=w481, "State"=w479, "Relay # (1=1st relay)"=16) -> ("Relay States OUT"=w480:bool[])  [unwired: 8 in]
                                n314 = local write "Relay States"(w480) -> ()
                                }
                                frame #4 {
                                n315 = Wait (ms)(milliseconds to wait=u32 2000) -> ()  [unwired: 1 out]
                                }
                              }
                            }
                          }
                        }
                      }
                    }
                    frame #2 {
                      "Countdown (secs)" <- w486
                    }
                  }
                  n316 = Wait (ms)(milliseconds to wait=u32 100) -> ()  [unwired: 1 out]
                }
              }
            }
          }
        }
      }
    }
    n317 = local read "stop"() -> (w363:bool)
  }
